vi "ConvertMeasureToUnitValue2.vi"(0 "input":dbl=1e-18 format="%#_6f", 1 "Frefix":T1(ring)=enum."nano", 2 "Unit":string="m", 3 "Format":string="%0.3f") -> (7 "output":string="0.825a", 8 "Raito":dbl=0.8250443524689961 format="%#_6p")   [LabVIEW 2018, in "Library-DataConvert.lvlib"]
uses:
  Library-DataConvert.lvlib
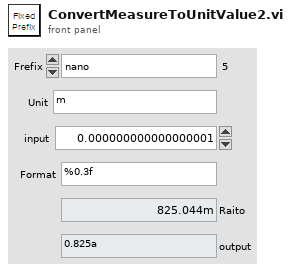
[diagram p1: front panel]
types:
  T1 = enum16{"yocto", "zepto", "atto", "femto", "pico", "nano", "micro", "milli", "centi", "deci", "1", "deca", "hecto", "kilo", "mega", "giga", "tera", "peta", "exa", "zetta", "yotta"}
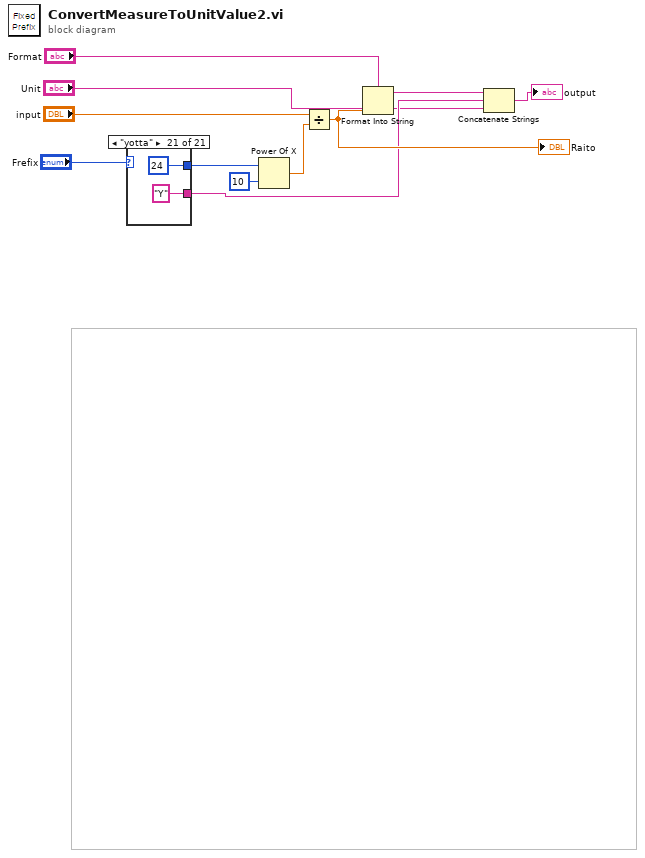
[diagram p0: block diagram]
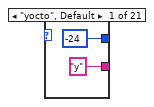
[diagram p2: hidden frame]
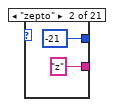
[diagram p3: hidden frame]
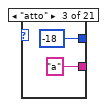
[diagram p4: hidden frame]
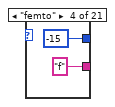
[diagram p5: hidden frame]
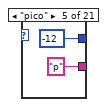
[diagram p6: hidden frame]
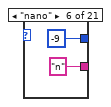
[diagram p7: hidden frame]
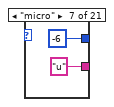
[diagram p8: hidden frame]
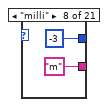
[diagram p9: hidden frame]
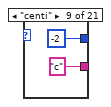
[diagram p10: hidden frame]
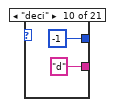
[diagram p11: hidden frame]
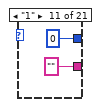
[diagram p12: hidden frame]
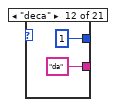
[diagram p13: hidden frame]
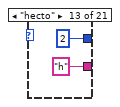
[diagram p14: hidden frame]
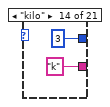
[diagram p15: hidden frame]
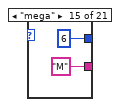
[diagram p16: hidden frame]
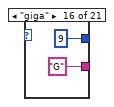
[diagram p17: hidden frame]
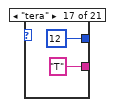
[diagram p18: hidden frame]
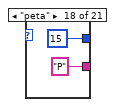
[diagram p19: hidden frame]
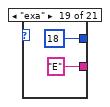
[diagram p20: hidden frame]
diagram:
  n1 = case shown="\"yotta\"" "Frefix" {
    tunnel: [-24 -21 -18 -15 -12 -9 -6 -3 -2 -1 0 1 2 3 6 9 12 15 18 21 24] -> w10
    tunnel: ["y" ("포맷 문자열") "z" ("포맷 문자열") "a" ("포맷 문자열") "f" ("포맷 문자열") "p" ("포맷 문자열") "n" ("포맷 문자열") "u" ("포맷 문자열") "m" ("포맷 문자열") "c" ("포맷 문자열") "d" ("포맷 문자열") "" ("포맷 문자열") "da" ("포맷 문자열") "h" ("포맷 문자열") "k" ("포맷 문자열") "M" ("포맷 문자열") "G" ("포맷 문자열") "T" ("포맷 문자열") "P" ("포맷 문자열") "E" ("포맷 문자열") "Z" ("포맷 문자열") "Y" ("포맷 문자열")] -> w3
    frame "yocto", Default {
    }
    frame "zepto" {
    }
    frame "atto" {
    }
    frame "femto" {
    }
    frame "pico" {
    }
    frame "nano" {
    }
    frame "micro" {
    }
    frame "milli" {
    }
    frame "centi" {
    }
    frame "deci" {
    }
    frame "1" {
    }
    frame "deca" {
    }
    frame "hecto" {
    }
    frame "kilo" {
    }
    frame "mega" {
    }
    frame "giga" {
    }
    frame "tera" {
    }
    frame "peta" {
    }
    frame "exa" {
    }
    frame "zetta" {
    }
    frame "yotta" {
    }
  }
  n2 = Power Of X(1:10 ("x"), 2:w10) -> (0:w8:dbl)
  n3 = Divide(x="input", y=w8) -> (x/y=w6:dbl)
  "Raito" <- w6
  n4 = Format Into String(format string="Format", w6) -> (resulting string=w5:string)  [unwired: 2 in, 1 out]
  n5 = Concatenate Strings(w5, w3, "Unit") -> (→"output":string)
